vi "Compute Max Level.vi"(0 "Waveform in":refnum<class "Waveform.lvclass">, 1 "Filter in":refnum<class "Filter.lvclass">, 5 "Level in":refnum<class "Level.lvclass">, 7 "Fs (Hz)":dbl, 9 "Vmax":dbl, 11 "error in (no error)":errorcluster) -> (4 "Waveform out":refnum<class "Waveform.lvclass">, 6 "Level thru":refnum<class "Level.lvclass">, 10 "Lmax":dbl, 15 "error out":errorcluster)   [LabVIEW 2020, in "Waveform.lvclass"]
uses:
  Waveform.lvclass
  Level/Level.lvclass
  Filter/Filter.lvclass
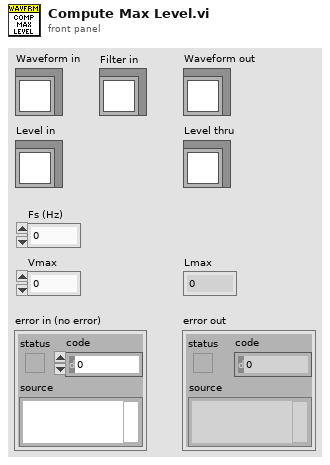
[diagram p1: front panel]
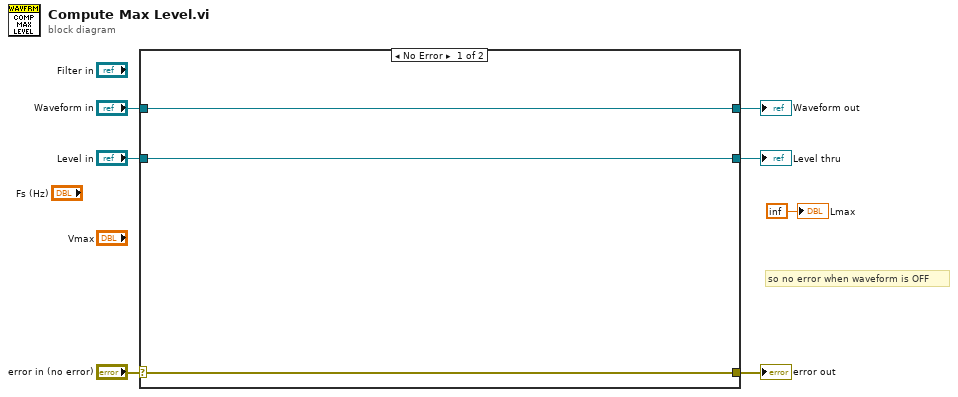
[diagram p0: block diagram]
diagram:
  # "so no error when waveform is OFF"
  n1 = case shown="No Error" "error in (no error)" {
    selector: "error in (no error)" -> [w9 w13]
    tunnel: [w9 w13] -> w6
    tunnel: [w10 w12] -> w4
    tunnel: "Waveform in" -> [w10 w12]
    tunnel: [w8 w11] -> w3
    tunnel: "Level in" -> [w8 w11]
    frame No Error {
    }
    frame Error {
    }
  }
  "error out" <- w6
  "Waveform out" <- w4
  "Level thru" <- w3
  "Lmax" <- inf
